vi "Compute Row Broken Streaks.vi"(11 "row map":string[](array[string])) -> (3 "broken streaks":u8[](array[numeric]))   [LabVIEW 2022 SP3]
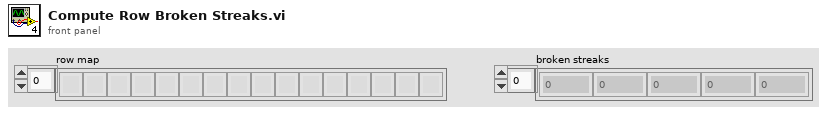
[diagram p1: front panel]
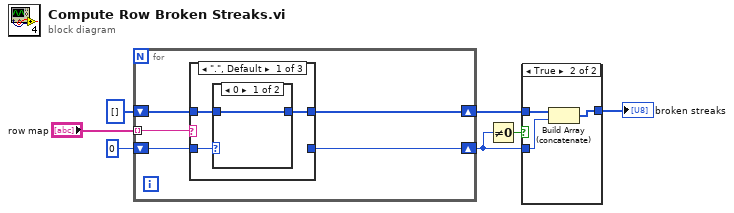
[diagram p0: block diagram]
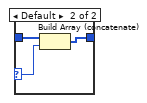
[diagram p3: hidden frame]
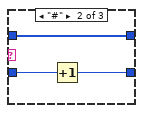
[diagram p4: hidden frame]
diagram:
  n1 = for {
    tunnel: "row map" -> [w12] mode=indexing
    shift-right: [w10] -> w3
    shift-left: u8 0 -> [w11]
    shift-right: [w9] -> w4
    shift-left: u8[] [] -> [w8]
    n2 = case shown="\".\", Default" w12 {
      tunnel: w11 -> [w15 w22 w24]
      tunnel: [_ w21 w24] -> w10
      tunnel: [w14 w20 w23] -> w9
      tunnel: w8 -> [w13 w20 w23]
      frame ".", Default {
        n3 = case shown="0" w15 {
          selector: w15 -> [_ w19]
          tunnel: [w16 w18] -> w14
          tunnel: w13 -> [w16 w17]
          frame 0 {
          }
          frame Default {
            n4 = Build Array (concatenate)(w17, w19) -> (w18:u8[])
          }
        }
      }
      frame "#" {
        n5 = Increment(x=w22) -> (x+1=w21:u8)
      }
      frame "?" {
      }
    }
  }
  n6 = Not Equal To 0?(x=w3) -> (x != 0?=w2:bool)
  n7 = case shown="True" w2 {
    tunnel: w4 -> [w25 w28]
    tunnel: w3 -> [_ w27]
    tunnel: [w25 w26] -> w1
    frame False {
    }
    frame True {
      n8 = Build Array (concatenate)(w28, w27) -> (w26:u8[])
    }
  }
  "broken streaks" <- w1
